vi "testApplicationRefnum.vi"() -> ()   [LabVIEW 2017, in "CodeCoverage.Tests.lvlib"]
uses:
  CodeCoverage.Tests.lvlib
  CodeCoverage/CodeCoverage.lvclass/CodeCoverage.ctl
  CodeCoverage/CodeCoverage.lvclass
  Assertion/Assertion.lvlib
panel:
  out "error out":errorcluster
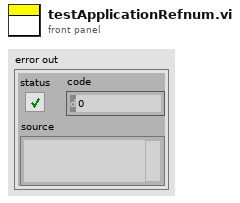
[diagram p1: front panel]
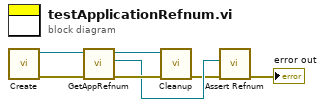
[diagram p0: block diagram]
diagram:
  n1 = call "Create.vi"() -> ("error out"=w6:errorcluster, "CodeCoverage out"=w7:refnum<class "CodeCoverage.lvclass">)  [unwired: 10 in]
  n2 = call "GetAppRefnum.vi"("error in (no error)"=w6, "CodeCoverage in"=w7) -> ("error out"=w4:errorcluster, "App Refnum"=w3:refnum<vi>, "CodeCoverage out"=w5:refnum<class "CodeCoverage.lvclass">)  [unwired: 7 in]
  n3 = call "Cleanup.vi"("error in (no error)"=w4, "CodeCoverage in"=w5) -> ("error out"=w2:errorcluster)  [unwired: 9 in]
  n4 = call "Assert Refnum.vi"("error in (no error)"=w2, "Refnum"=w3) -> ("error out"=→"error out":errorcluster)  [unwired: 9 in]
